vi "numeric to AuditHMI thread id enum.vi"(11 "Numeric":i32) -> (3 "Station cDAQ Thread Queues out":T1=enum."tcp comms")   [LabVIEW 2012]
uses:
  typedefs/station AuditHMI thread IDs.ctl
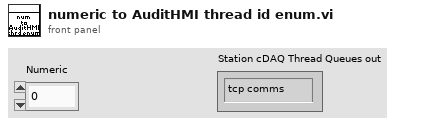
[diagram p1: front panel]
types:
  T1 = typedef "station AuditHMI thread IDs.ctl" = enum16{"AuditHMI main", "tcp comms"}
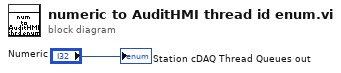
[diagram p0: block diagram]
diagram:
  "Station cDAQ Thread Queues out" <- "Numeric"
